vi "start FIFOs.vi"(8 "error in":errorcluster, 11 "profibus reference":T1) -> (0 "error out":errorcluster, 3 "profibus reference out":T1)   [LabVIEW 2013, in "dynamic profibus.lvlib"]
uses:
  dynamic profibus.lvlib
  fpga reference.ctl
  <vilib>/rvi/interface/common/niFpgaWaitOnOcc.vi
  <vilib>/Utility/error.llb/Error Cluster From Error Code.vi
  <vilib>/rvi/interface/nirviMethod/nirviMethod.xnode
  <vilib>/rvi/errors/niLvFpgaMergeErrorWithErrorCode.vi
  <vilib>/FPGAPlugInAG/Dynamic/niLvFpga_StartFifo_Dynamic.vi
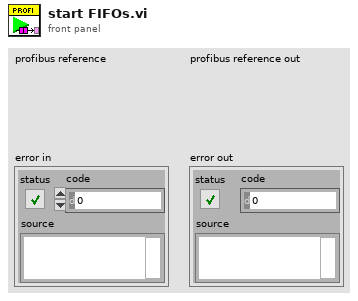
[diagram p1: front panel]
types:
  T1 = typedef "dynamic profibus.lvlib/fpga reference.ctl" = refnum<k20>
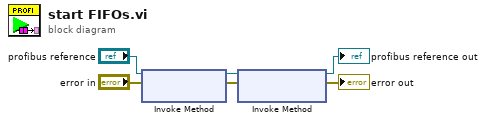
[diagram p0: block diagram]
diagram:
  n1 = xnode "Invoke Method"("FPGA VI Reference In"="profibus reference", "error in"="error in") -> ("FPGA VI Reference Out"=w2:T1, "error out"=w5:errorcluster)
  n2 = xnode "Invoke Method"("FPGA VI Reference In"=w2, "error in"=w5) -> ("FPGA VI Reference Out"=→"profibus reference out":T1, "error out"=→"error out":errorcluster)
